vi "opencvTest.vi"() -> ()   [LabVIEW 2017]
uses:
  opencv/build/x64/vc15/bin/opencv_world341.dll
panel:
  out "Waveform Graph 2":u16[][](graph)
  out "Waveform Graph":u16[][](graph)
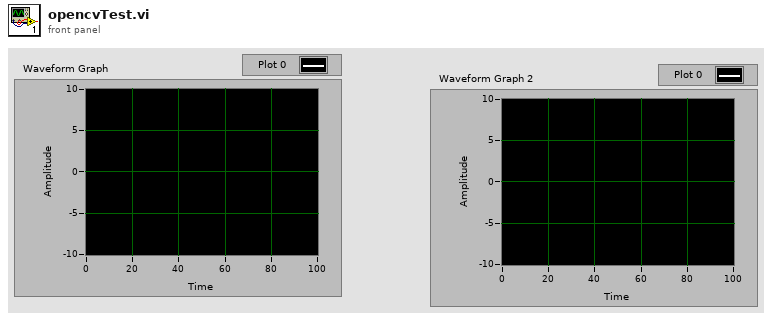
[diagram p1: front panel]
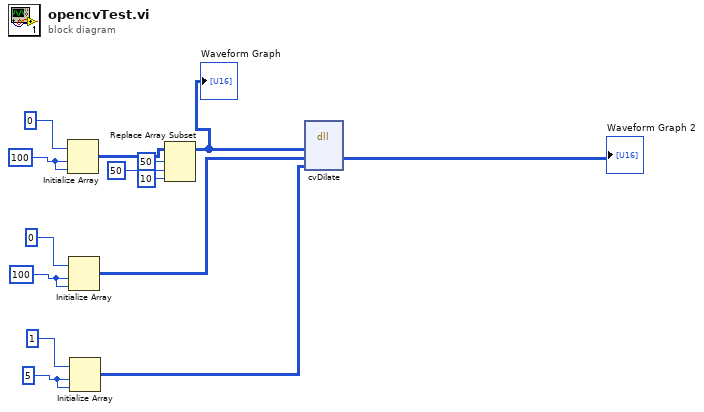
[diagram p0: block diagram]
diagram:
  w4 = 5 ("dimension size")
  w8 = 100 ("dimension size")
  w13 = 100 ("dimension size")
  n1 = Initialize Array(u16 0 ("element"), w13, w13) -> (w12:u16[][])
  n2 = Initialize Array(u16 0 ("element"), w8, w8) -> (w6:u16[][])
  n3 = Initialize Array(u16 1 ("element"), w4, w4) -> (w3:u16[][])
  n4 = Replace Array Subset(array=w12, new element=u16 10 ("new element/subarray"), index (row)=50, index (col)=50 ("disabled index (col)")) -> (w2:u16[][])
  "Waveform Graph" <- w2
  n5 = dll-call lib="C:/Users/francesco/dev/pump-probe/opencv/build/x64/vc15/bin/opencv_world341.dll" fn="cvDilate"("src"=w2, "dst"=w6, "kernel"=w3) -> ("dst"=→"Waveform Graph 2":u16[][])  [unwired: 6 in, 2 out]
